vi "Config Variant.vi"(10 "Count":path=path "D:/Data Actuator/config/Settings", 11 "test sequence":path=path "D:/Data Actuator/config/Settings") -> ()   [LabVIEW 2023]
uses:
  test setting.ctl
panel:
  in  "Path For Laser File":path
  in  "Next Barcode Printing Wait Time":i32 caption="Next Barcode Printing\nWait Time (Sec.)"
  in  "Part Identification Code":string="02BABCD1009190487LKWPG"
  in  "Vendor Code":string="02BABCD1009190487LKWPG"
  in  "M&M Part No.":string="02BABCD1009190487LKWPG"
  in  "MODEL NAME":string(combo)
  in  "Add":bool
  in  "Delete":bool
  in  "Save Model":bool
  in  "Exit":bool
  out "error out":errorcluster
  out "connection ID Out":refnum<k5>
  in  "error in":errorcluster
  in  "connection ID in":refnum<k5>
  out "AI38 2":bool
  out "Stop Button":bool
  # "COLLER LEAK TESTING DATALOGGING SYSTEM"
  # "RECIPE SCREEN"
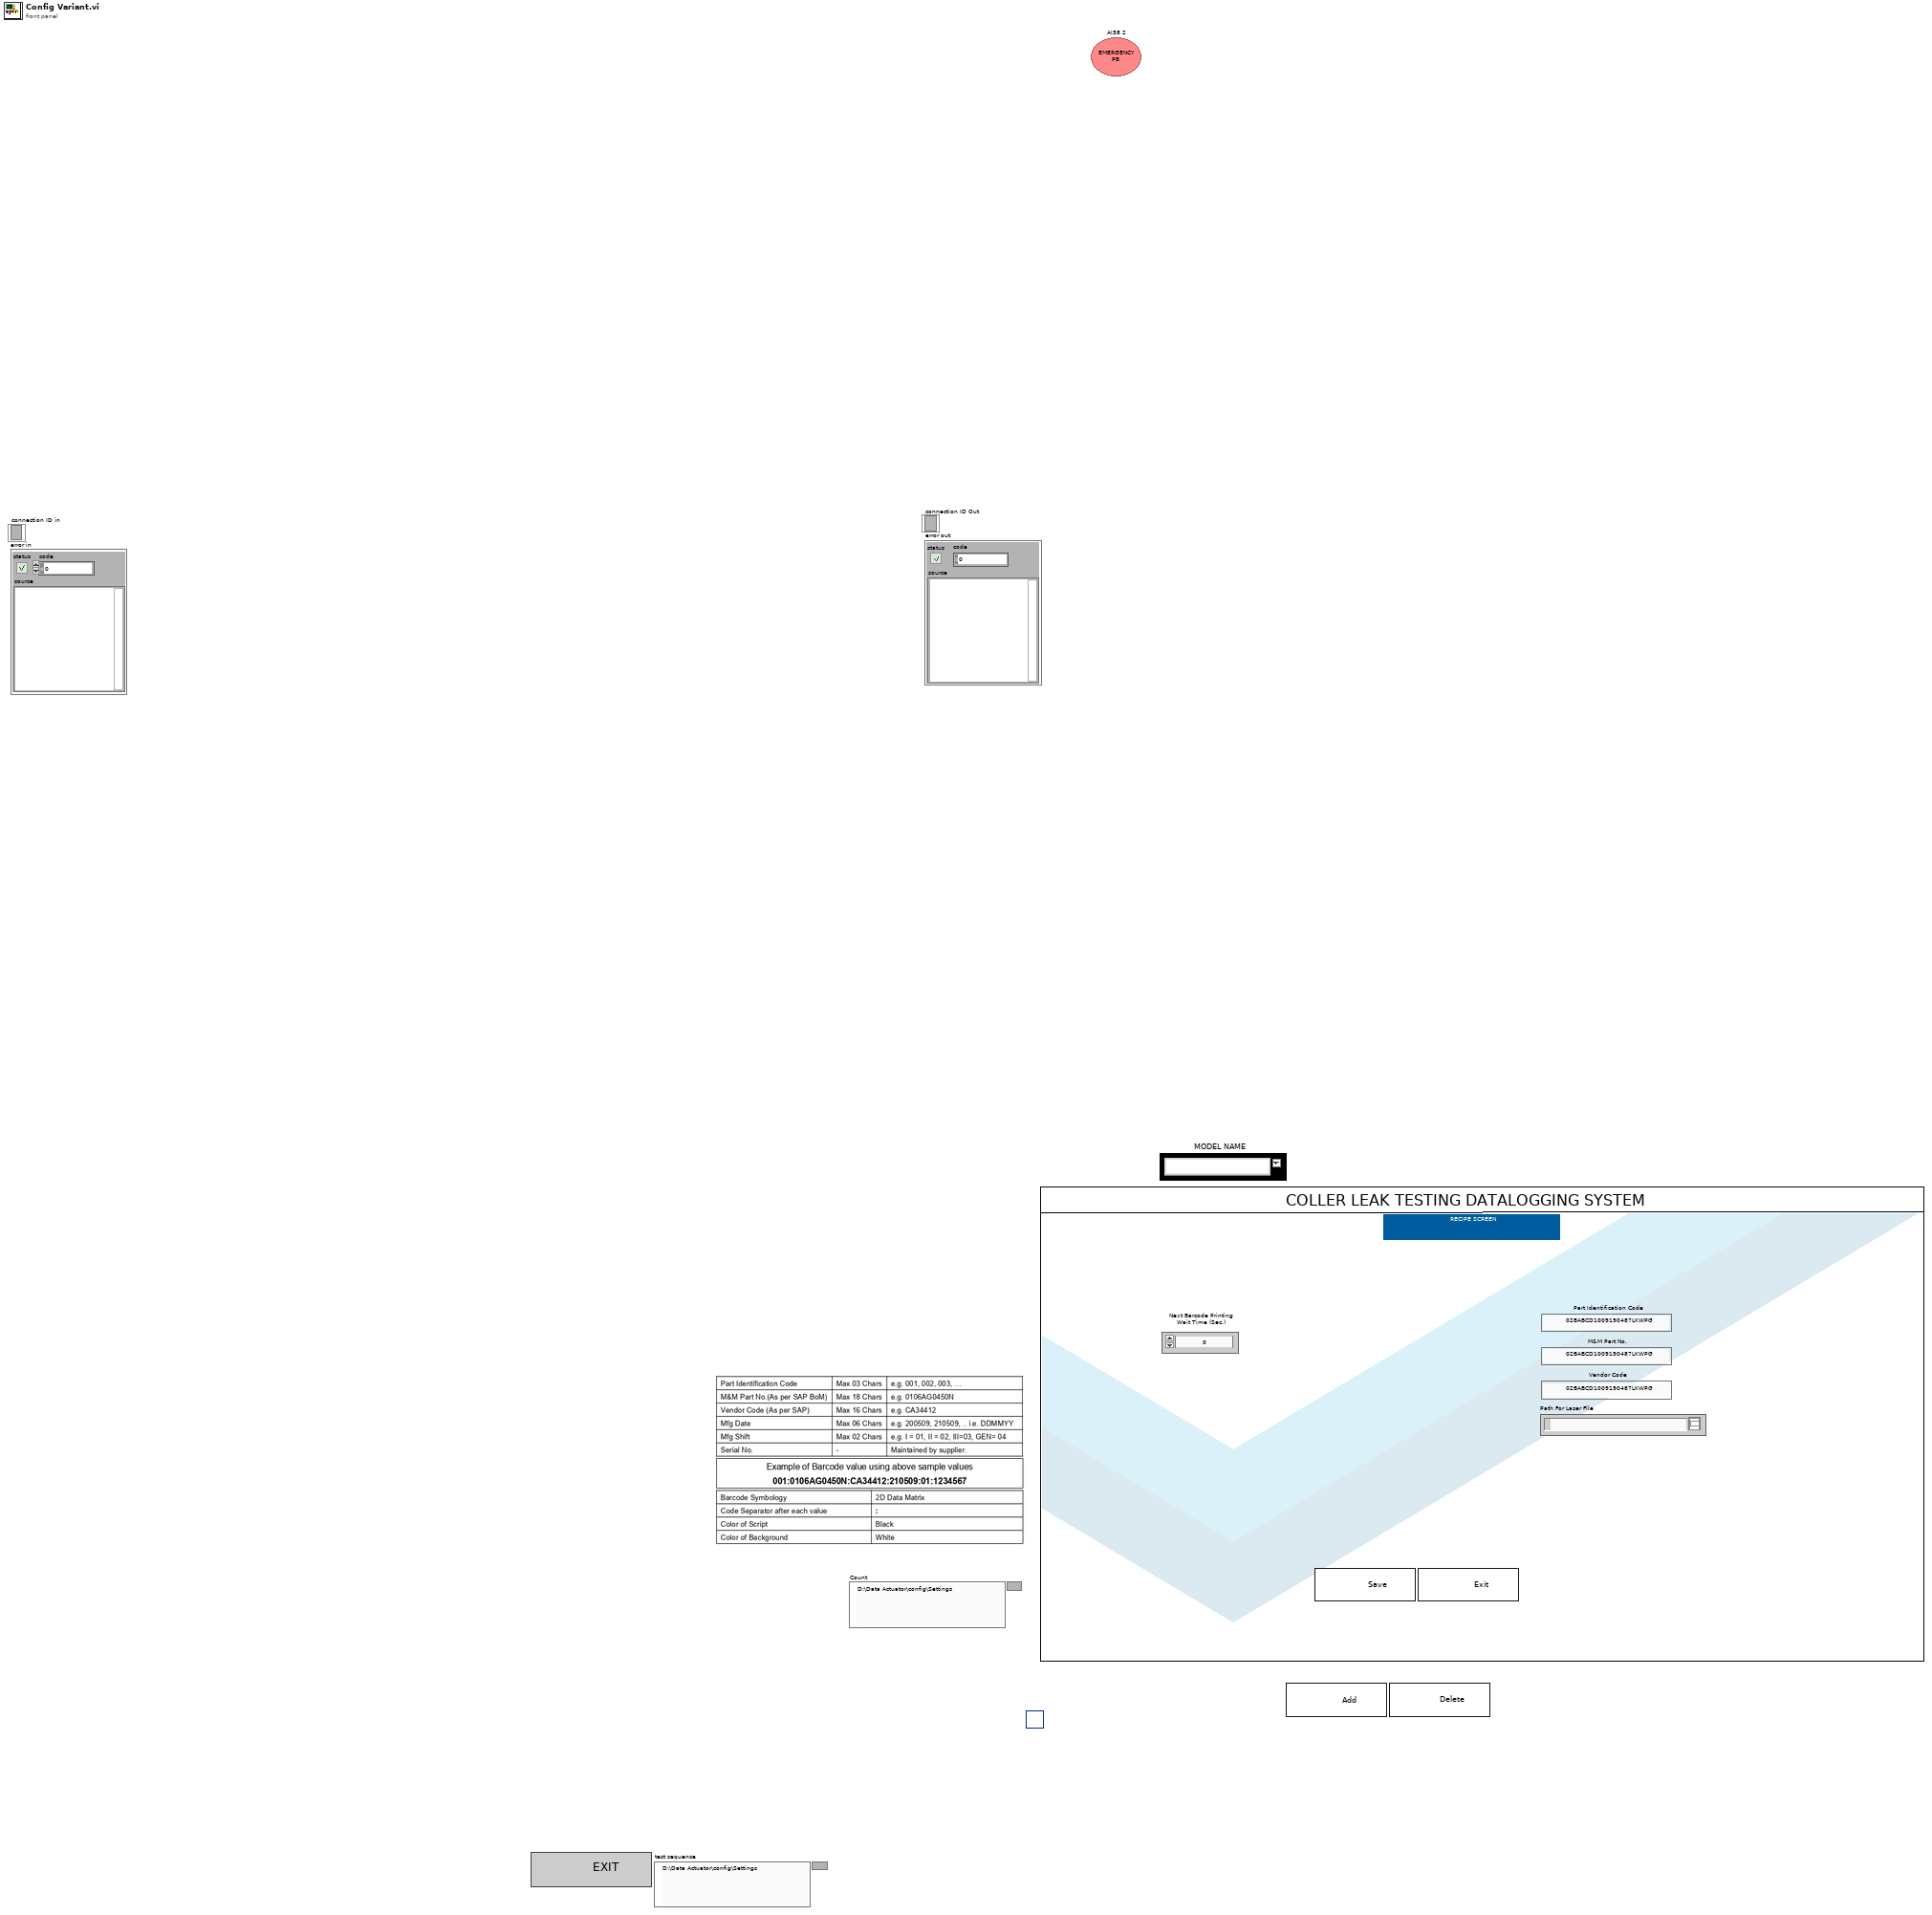
[diagram p1: front panel]
types:
  T1 = typedef "test setting.ctl" = cluster{"M&M Part No.":string, "Vendor Code":string, "Part Identification Code":string, "Next Barcode Printing Wait Time":i32, "Path for LAser":path}
  T2 = enum16{"open", "replace", "create", "open or create", "replace or create", "replace or create with confirmation"}
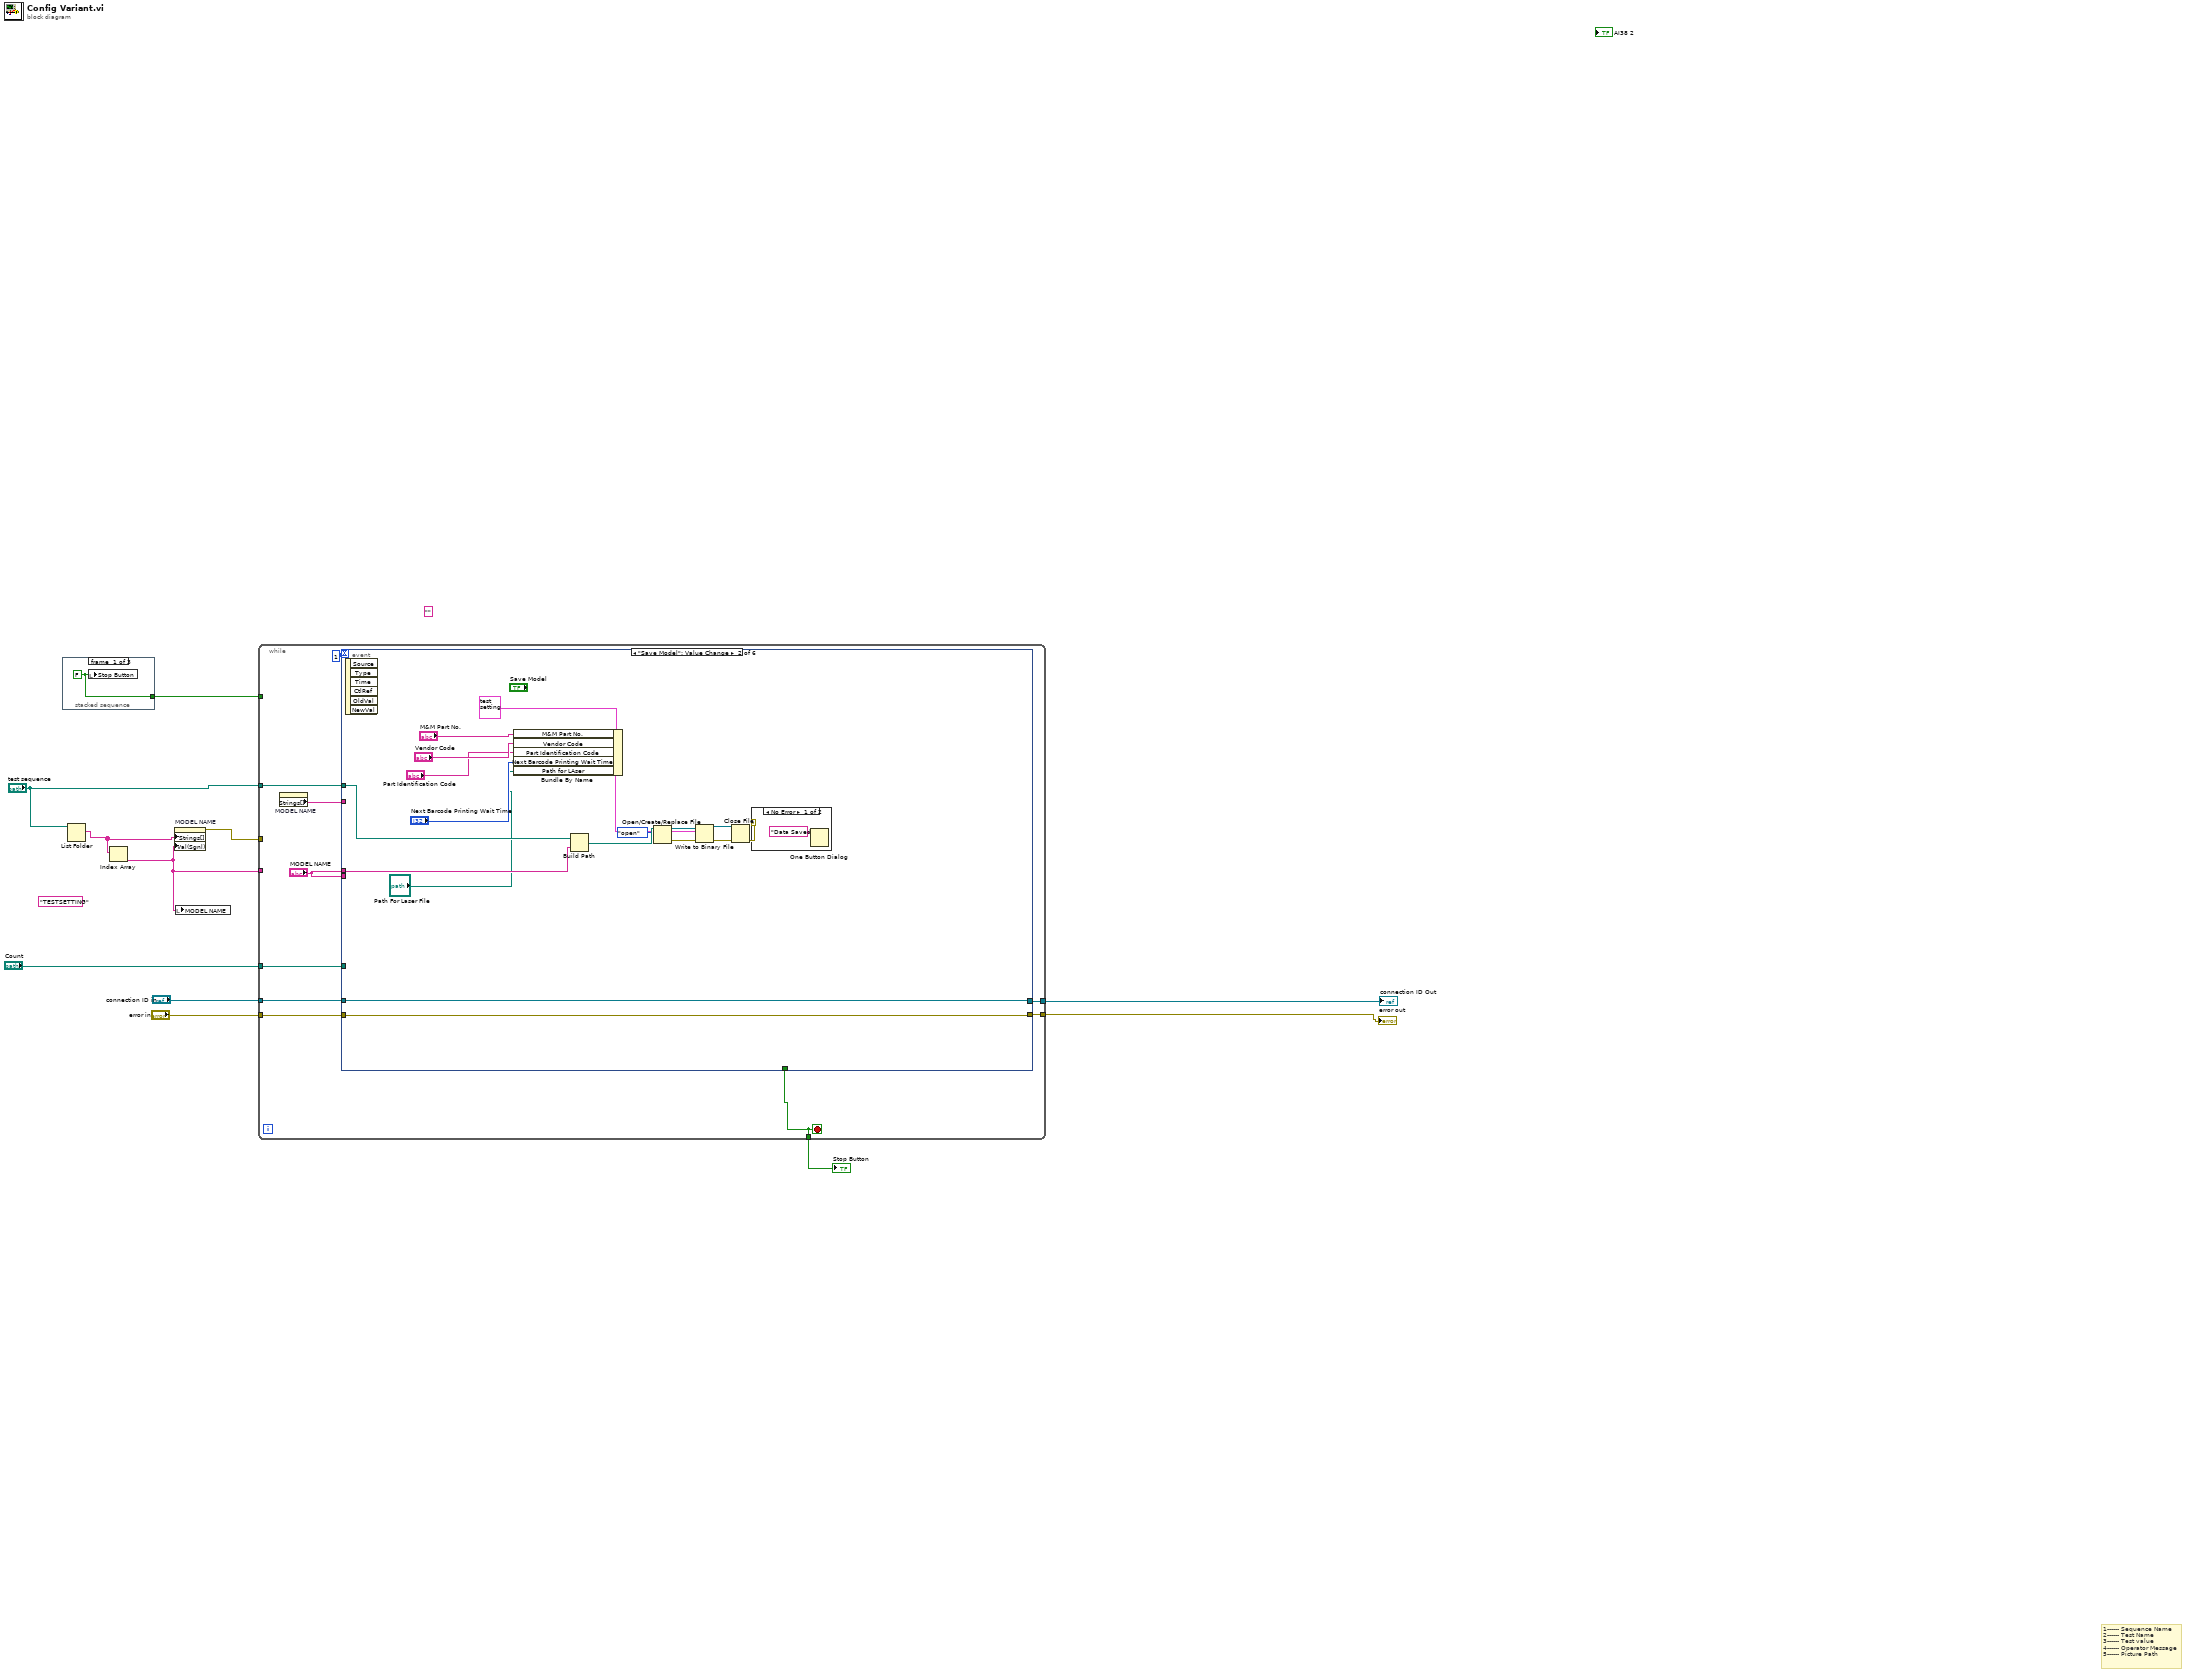
[diagram p0: block diagram]
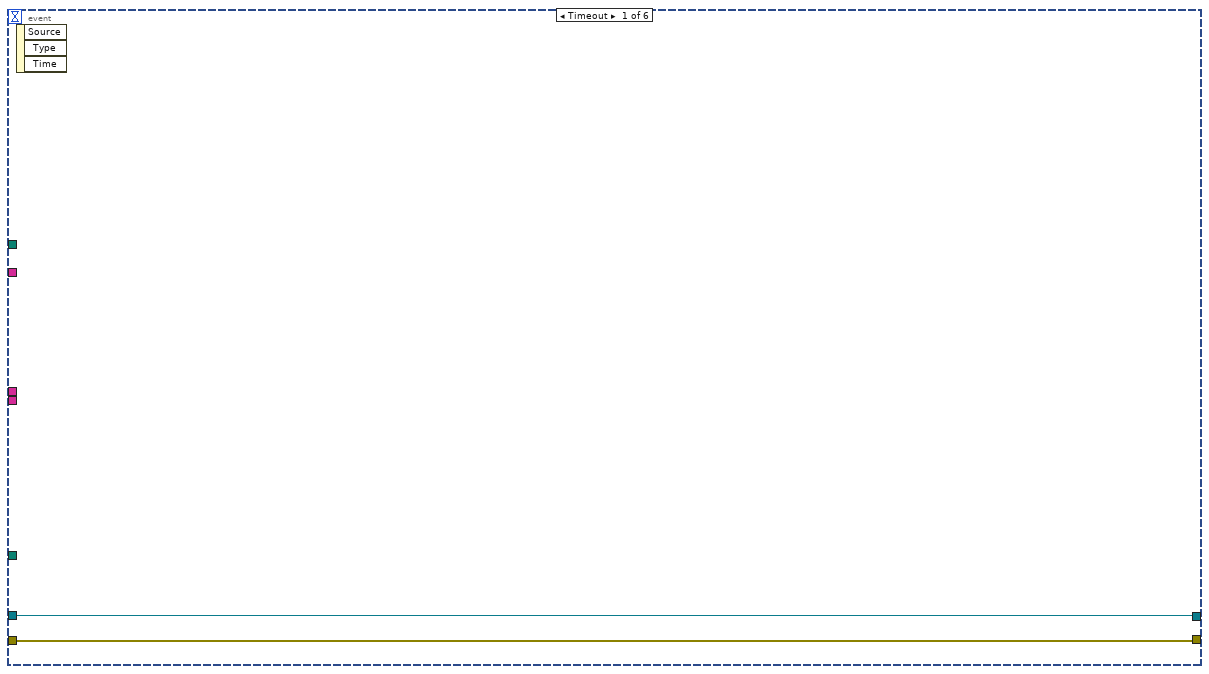
[diagram p4: hidden frame]
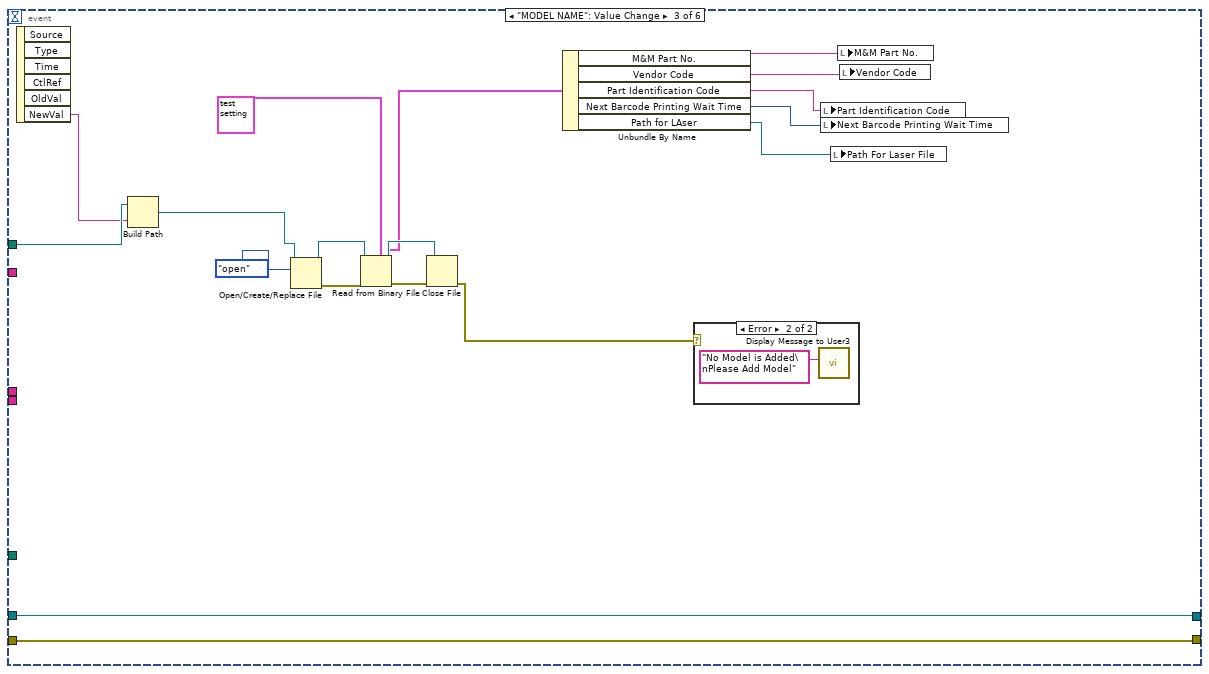
[diagram p6: hidden frame]
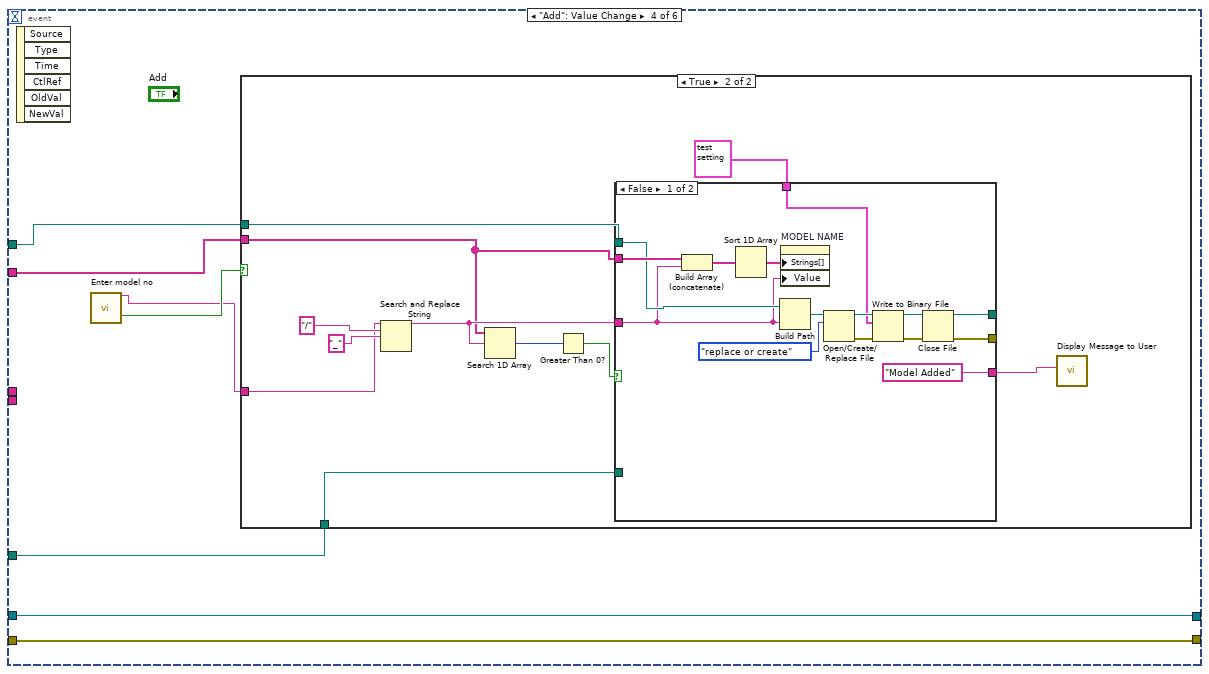
[diagram p8: hidden frame]
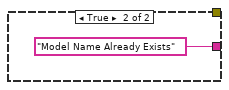
[diagram p10: hidden frame]
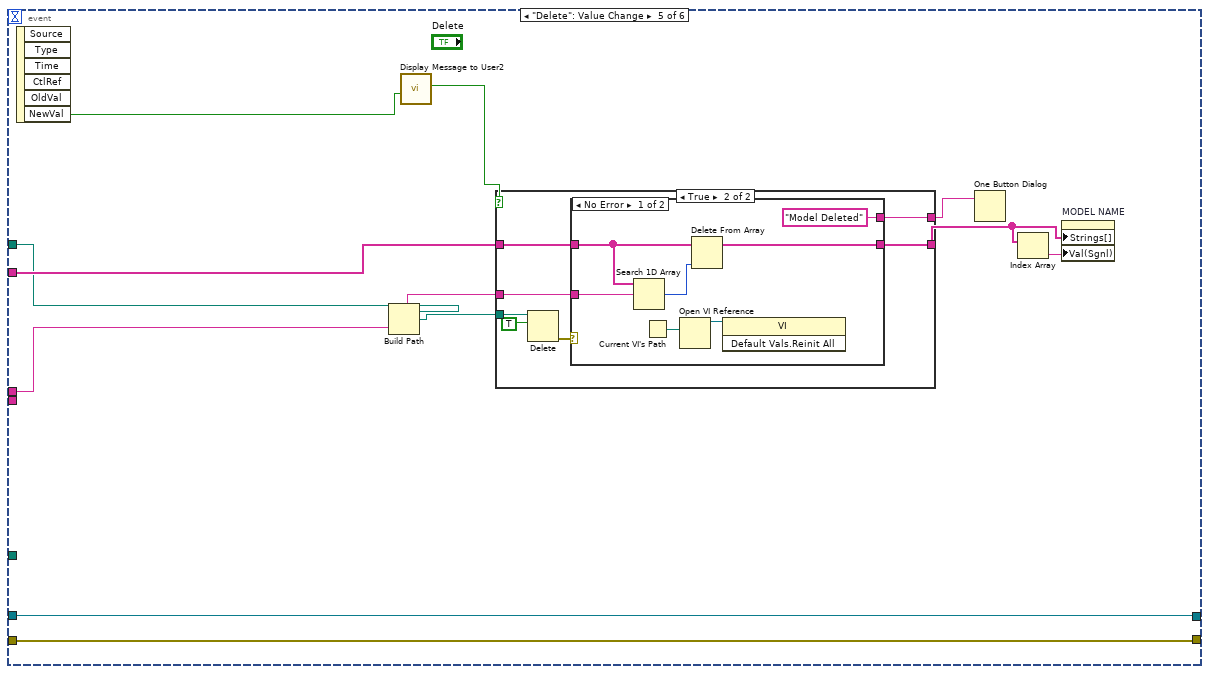
[diagram p11: hidden frame]
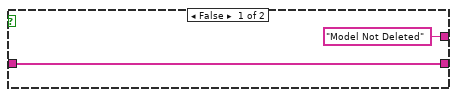
[diagram p12: hidden frame]
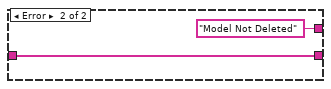
[diagram p13: hidden frame]
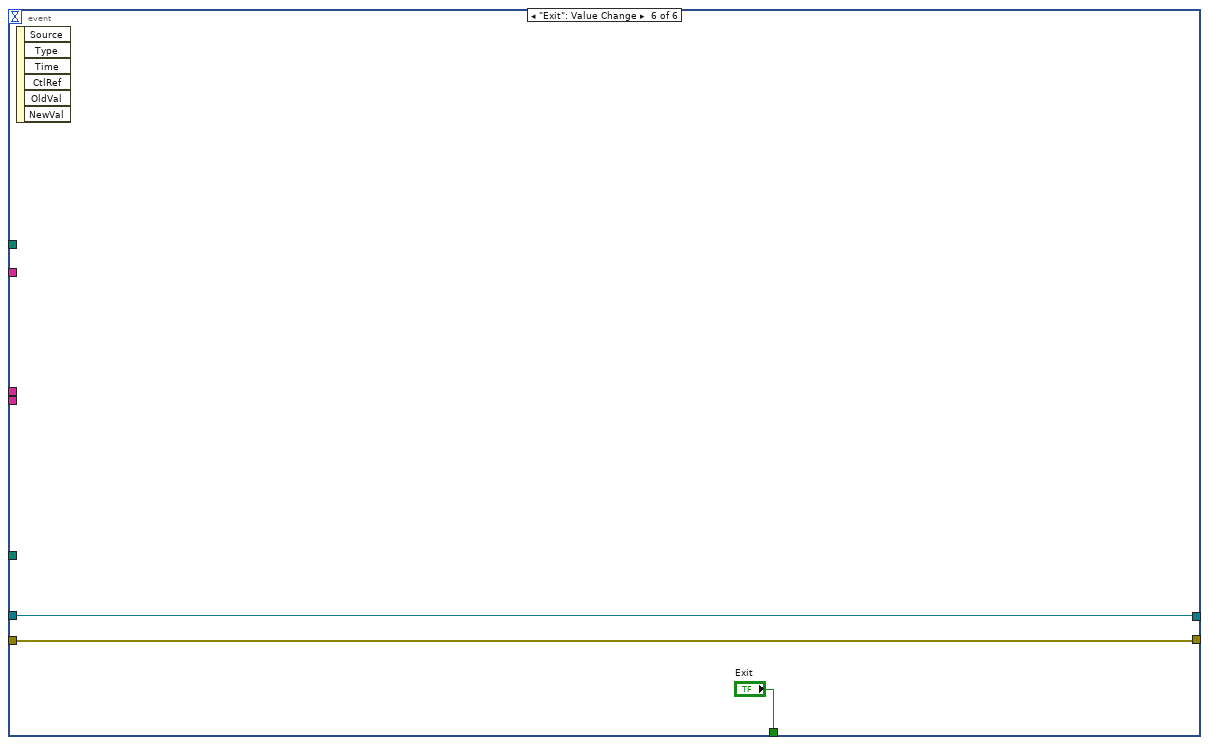
[diagram p14: hidden frame]
diagram:
  (unwired) "" ("ENGINE BARCODE PREFIX")
  (unwired) "TESTSETTING" ("Value (Signaling)")
  # "1------ Sequence Name\n2------ Test Name\n3------ Test value\n4------ Operator Message\n5------ Picture Path"
  n1 = stacked-sequence {
    tunnel: [w12 _ _] -> w4
    frame #0 {
      w12 = FALSE ("Stop Button")
      n2 = local write "Stop Button"(w12) -> ()
    }
    frame #1 {
    }
    frame #2 {
    }
  }
  n3 = List Folder(path="test sequence") -> (filenames=w3:string[])  [unwired: 3 in, 3 out]
  n4 = Index Array(array=w3) -> (element=w2:string)  [unwired: 1 in]
  n5 = property on="MODEL NAME" class="CmbBox"("Strings[]"=w3, "Val(Sgnl)"=w2) -> (error out=w9:errorcluster)  [unwired: 2 in, 1 out]
  n6 = local write "MODEL NAME"(w2) -> ()
  n7 = while {
    tunnel: "test sequence" -> [w21]
    tunnel: [w19] -> w10
    tunnel: w2 -> [_]
    tunnel: w9 -> [_]
    tunnel: "connection ID in" -> [w17]
    tunnel: "error in" -> [w16]
    tunnel: [w15] -> w6
    tunnel: [w14] -> w5
    tunnel: w4 -> [_]
    tunnel: "Count" -> [w13]
    stop <- w19 stop-if-true
    n8 = property on="MODEL NAME" class="CmbBox"() -> ("Strings[]"=w20:string[])  [unwired: 2 in, 2 out]
    n9 = event shown="[1] \"Save Model\": Value Change" {
      selector: _ -> [_ _ _ _ _ _]
      dyn-events: _ -> [_ _ _ _ _ _]
      timeout: 1 -> [_ _ _ _ _ _]
      tunnel: w21 -> [_ w35 w52 w68 w101 _]
      tunnel: "MODEL NAME" -> [_ _ _ _ _ _]
      tunnel: w20 -> [_ _ _ w69 w102 _]
      tunnel: [_ _ _ _ _ "Exit"] -> w19
      tunnel: "MODEL NAME" -> [_ w34 _ _ w99 _]
      tunnel: w17 -> [w24 w32 w51 w66 w98 w127]
      tunnel: w16 -> [w23 w31 w50 w65 w97 w126]
      tunnel: [w24 w32 w51 w66 w98 w127] -> w15
      tunnel: [w23 w31 w50 w65 w97 w126] -> w14
      tunnel: w13 -> [_ _ _ w63 _ _]
      event Timeout {
        n10 = event-data() -> ()  [unwired: 1 in, 3 out]
      }
      event "Save Model": Value Change {
        n11 = event-data() -> ()  [unwired: 1 in, 6 out]
        n12 = Bundle By Name(cluster=T1 {"M&M Part No."="", "Vendor Code"="02BHMSI1009190338RKWPG", "Part Identification Code"="02CRMTT1009190250KWPG", "Next Barcode Printing Wait Time"=0, "Path for LAser"=path ""} ("Cluster"), "M&M Part No."="M&M Part No.", "Vendor Code"="Vendor Code", "Part Identification Code"="Part Identification Code", "Next Barcode Printing Wait Time"="Next Barcode Printing Wait Time", "Path for LAser"="Path For Laser File") -> (w30:T1)
        n13 = Build Path(base path=w35, name or relative path=w34) -> (appended path=w41:path)
        n14 = Open/Create/Replace File(file path (use dialog)=w41, operation (0:open)=T2."open") -> (refnum out=w37:refnum<file>, error out=w40:errorcluster)  [unwired: 4 in, 1 out]
        n15 = Write to Binary File(file (use dialog)=w37, data=w30, error in=w40) -> (refnum out=w38:refnum<file>, error out=w39:errorcluster)  [unwired: 3 in, 1 out]
        n16 = Close File(refnum=w38, error in=w39) -> (error out=w42:errorcluster)  [unwired: 1 out]
        n17 = case shown="No Error" w42 {
          frame No Error {
            n18 = One Button Dialog(message="Data Saved") -> ()  [unwired: 1 in, 1 out]
          }
          frame Error {
          }
        }
      }
      event "MODEL NAME": Value Change {
        n19 = event-data() -> ("NewVal"=w49:string)  [unwired: 1 in, 5 out]
        n20 = Build Path(base path=w52, name or relative path=w49) -> (appended path=w56:path)
        n21 = Open/Create/Replace File(file path (use dialog)=w56, operation (0:open)=T2."open") -> (refnum out=w57:refnum<file>, error out=w58:errorcluster)  [unwired: 4 in, 1 out]
        n22 = Read from Binary File(5:T1 {"M&M Part No."="", "Vendor Code"="02BHMSI1009190338RKWPG", "Part Identification Code"="02CRMTT1009190250KWPG", "Next Barcode Printing Wait Time"=0, "Path for LAser"=path ""} ("Cluster"), 8:w58, 11:w57) -> (0:w60:errorcluster, 2:w53:T1, 3:w59:refnum<file>)  [unwired: 3 in, 1 out]
        n23 = Close File(refnum=w59, error in=w60) -> (error out=w55:errorcluster)  [unwired: 1 out]
        n24 = Unbundle By Name(w53) -> ("M&M Part No."=w48:string, "Vendor Code"=w47:string, "Part Identification Code"=w46:string, "Next Barcode Printing Wait Time"=w45:i32, "Path for LAser"=w44:path)
        n25 = case shown="Error" w55 {
          frame No Error {
          }
          frame Error {
            n26 = call "Display Message to User3"("Message"="No Model is Added\nPlease Add Model") -> ()  [unwired: 9 in, 2 out]
          }
        }
        n27 = local write "Part Identification Code"(w46) -> ()
        n28 = local write "Next Barcode Printing Wait Time"(w45) -> ()
        n29 = local write "Path For Laser File"(w44) -> ()
        n30 = local write "M&M Part No."(w48) -> ()
        n31 = local write "Vendor Code"(w47) -> ()
      }
      event "Add": Value Change {
        n32 = event-data() -> ()  [unwired: 1 in, 6 out]
        n33 = call "Enter model no.vi"() -> ("decimal integer string"=w64:string, "OK"=w67:bool)  [unwired: 17 in, 1 out]
        n34 = case shown="True" w67 {
          tunnel: w69 -> [_ w70]
          tunnel: w68 -> [_ w73]
          tunnel: w64 -> [_ w72]
          tunnel: w63 -> [_ w71]
          frame False {
          }
          frame True {
            n35 = Search and Replace String(input string=w72, search string="/", replace string="_" ("replace string (\"\")")) -> (result string=w79:string)  [unwired: 5 in, 3 out]
            n36 = Search 1D Array(1D array=w70, element=w79) -> (index of element=w74:i32)  [unwired: 1 in]
            n37 = Greater Than 0?(x=w74) -> (x > 0?=w75:bool)
            n38 = case shown="False" w75 {
              tunnel: ["Model Added" "Model Name Already Exists"] -> w76
              tunnel: w70 -> [w95 _]
              tunnel: w79 -> [w81 _]
              tunnel: [w85 _] -> _
              tunnel: T1 {"M&M Part No."="", "Vendor Code"="02BHMSI1009190338RKWPG", "Part Identification Code"="02CRMTT1009190250KWPG", "Next Barcode Printing Wait Time"=0, "Path for LAser"=path ""} ("Cluster") -> [w84 _]
              tunnel: w73 -> [w83 _]
              tunnel: [w82 _] -> _
              tunnel: w71 -> [_ _]
              frame False {
                n39 = Build Array (concatenate)(w95, w81) -> (w88:string[])
                n40 = Sort 1D Array(array=w88) -> (sorted array=w87:string[])
                n41 = Build Path(base path=w83, name or relative path=w81) -> (appended path=w93:path)
                n42 = property on="MODEL NAME" class="CmbBox"("Strings[]"=w87, "Value"=w81) -> ()  [unwired: 2 in, 2 out]
                n43 = Open/Create/Replace File(file path (use dialog)=w93, operation (0:open)=T2."replace or create") -> (refnum out=w94:refnum<file>, error out=w91:errorcluster)  [unwired: 4 in, 1 out]
                n44 = Write to Binary File(file (use dialog)=w94, data=w84, error in=w91) -> (refnum out=w90:refnum<file>, error out=w89:errorcluster)  [unwired: 3 in, 1 out]
                n45 = Close File(refnum=w90, error in=w89) -> (path=w85:path, error out=w82:errorcluster)
              }
              frame True {
              }
            }
            n46 = call "Display Message to User"("Message"=w76) -> ()  [unwired: 9 in, 2 out]
          }
        }
      }
      event "Delete": Value Change {
        n47 = event-data() -> ("NewVal"=w100:bool)  [unwired: 1 in, 5 out]
        n48 = Build Path(base path=w101, name or relative path=w99) -> (appended path=w104:path)
        n49 = call "Display Message to User2"("Enable"=w100) -> ("OK"=w103:bool)  [unwired: 9 in, 1 out]
        n50 = case shown="True" w103 {
          tunnel: w104 -> [_ w116]
          tunnel: ["Model Not Deleted" w111] -> w105
          tunnel: [w108 w112] -> w106
          tunnel: w102 -> [w108 w113]
          tunnel: w99 -> [_ w110]
          frame False {
          }
          frame True {
            n51 = Delete(path (use dialog)=w116, entire hierarchy (F)=TRUE) -> (error out=w114:errorcluster)  [unwired: 3 in, 2 out]
            n52 = case shown="No Error" w114 {
              tunnel: w113 -> [w121 w125]
              tunnel: w110 -> [w123 _]
              tunnel: [w120 w125] -> w112
              tunnel: ["Model Deleted" "Model Not Deleted"] -> w111
              frame No Error {
                n53 = Search 1D Array(1D array=w121, element=w123) -> (index of element=w122:i32)  [unwired: 1 in]
                n54 = Current VI's Path() -> (path=w118:path)
                n55 = Open VI Reference(vi path=w118) -> (vi reference=w117:refnum<vi>)  [unwired: 5 in, 1 out]
                n56 = Delete From Array(array=w121, index=w122) -> (array with subset deleted=w120:string[])  [unwired: 1 in, 1 out]
                n57 = invoke class="VI" method="Default Vals.Reinit All"(reference=w117) -> ()  [unwired: 2 in, 3 out]
              }
              frame Error {
              }
            }
          }
        }
        n58 = One Button Dialog(message=w105) -> ()  [unwired: 1 in, 1 out]
        n59 = Index Array(array=w106) -> (element=w107:string)  [unwired: 1 in]
        n60 = property on="MODEL NAME" class="CmbBox"("Strings[]"=w106, "Val(Sgnl)"=w107) -> ()  [unwired: 2 in, 2 out]
      }
      event "Exit": Value Change {
        n61 = event-data() -> ()  [unwired: 1 in, 6 out]
      }
    }
  }
  "Stop Button" <- w10
  "connection ID Out" <- w6
  "error out" <- w5
